vi "as2_writeLogEntry.vi"(0 "Path In":path, 1 "Curr Param":dbl[](array[numeric])=[0.0, 3.0, 0.2, 1.0, 500.0] caption="Current Parameters", 2 "error in (no error)":errorcluster) -> (6 "error out":errorcluster)   [LabVIEW 2013]
uses:
  <vilib>/Utility/file.llb/Write To Spreadsheet File (string).vi
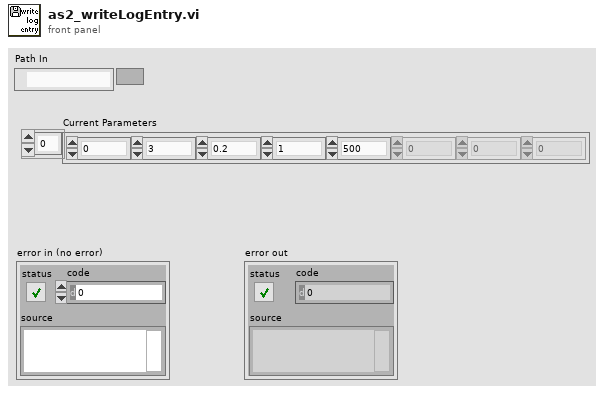
[diagram p1: front panel]
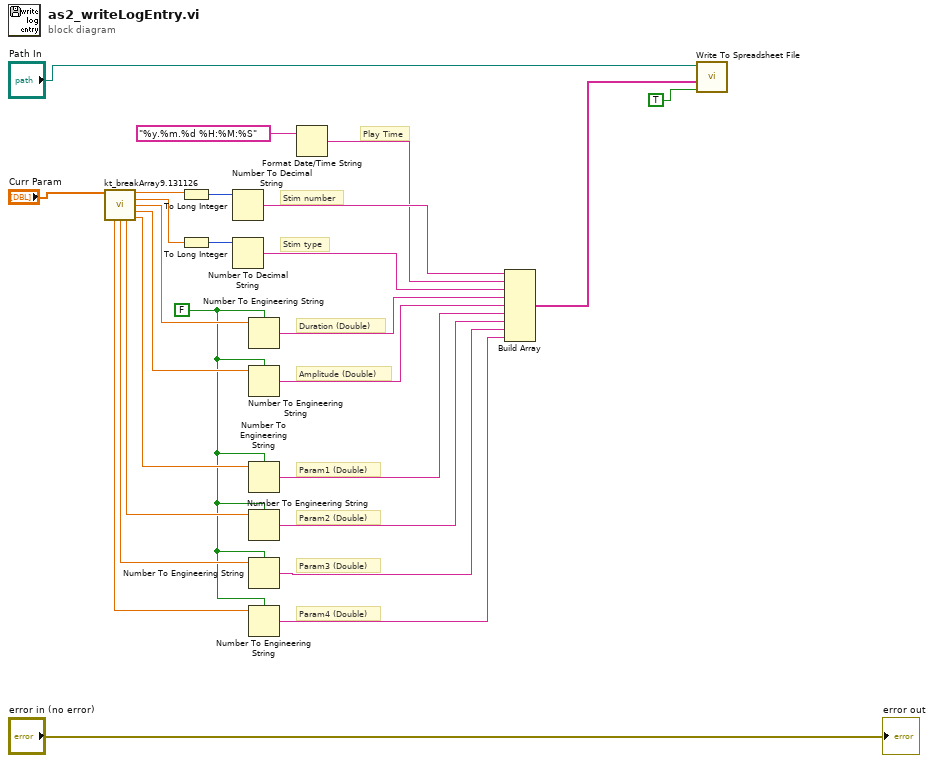
[diagram p0: block diagram]
diagram:
  w5 = FALSE ("use system decimal point (T)")
  # "Param4 (Double)"
  # "Param3 (Double)"
  # "Param2 (Double)"
  # "Param1 (Double)"
  # "Stim type"
  # "Amplitude (Double)"
  # "Duration (Double)"
  # "Play Time"
  # "Stim number"
  n1 = call "kt_breakArray9.131126.vi"("Current (or Cued Trial Parameters)"="Curr Param") -> ("Value 0"=w21:dbl, "Value 1"=w15:dbl, "Value 2"=w14:dbl, "Value 3"=w18:dbl, "Value 7"=w6:dbl, "Value 6"=w7:dbl, "Value 5"=w8:dbl, "Value 4"=w13:dbl)  [unwired: 6 in, 1 out]
  n2 = To Long Integer(number=w21) -> (32bit integer=w22:i32)
  n3 = To Long Integer(number=w15) -> (32bit integer=w17:i32)
  n4 = Number To Decimal String(number=w22) -> (decimal integer string=w20:string)  [unwired: 1 in]
  n5 = Number To Decimal String(number=w17) -> (decimal integer string=w16:string)  [unwired: 1 in]
  n6 = Number To Engineering String(1:w5, 4:w14) -> (0:w12:string)  [unwired: 2 in]
  n7 = Number To Engineering String(1:w5, 4:w18) -> (0:w11:string)  [unwired: 2 in]
  n8 = Number To Engineering String(1:w5, 4:w13) -> (0:w3:string)  [unwired: 2 in]
  n9 = Number To Engineering String(1:w5, 4:w8) -> (0:w4:string)  [unwired: 2 in]
  n10 = Number To Engineering String(1:w5, 4:w7) -> (0:w2:string)  [unwired: 2 in]
  n11 = Number To Engineering String(1:w5, 4:w6) -> (0:w1:string)  [unwired: 2 in]
  n12 = Format Date/Time String(time format string (%c)="%y.%m.%d %H:%M:%S") -> (date/time string=w19:string)  [unwired: 2 in]
  n13 = Build Array(w20, w19, w16, w12, w11, w3, w4, w2, w1) -> (w9:string[])
  n14 = call-poly <vilib>:"Write To Spreadsheet File.vi"("append to file? (new file:F)"=TRUE, "1D data"=w9, "file path (dialog if empty)"="Path In") -> ()  [unwired: 5 in, 1 out]
  "error out" <- "error in (no error)"
